vi "Drive Until Loss of Vision.vi"(11 "Distance Setpoint":dbl=56.0) -> (3 "ready to approach":bool=TRUE)   [LabVIEW 2016]
uses:
  Robot Values.vi
  Vision Global.vi
  <vilib>/addons/control/pid/pid.llb/PID (DBL).vi
  <vilib>/addons/control/pid/NI_PID_pid.lvlib
panel:
  in  "Baseline Power":dbl=0.5
  in  "Vision PID Gains":T1={"proportional gain (Kc)"=0.65, "integral time (Ti, min)"=0.0, "derivative time (Td, min)"=0.0} {"derivative time (Td, min)" format="%.3f"; "integral time (Ti, min)" format="%.3f"; "proportional gain (Kc)" format="%.3f"}
  in  "PID gains":T1={"proportional gain (Kc)"=1.0, "integral time (Ti, min)"=0.01, "derivative time (Td, min)"=0.0} {"derivative time (Td, min)" format="%.3f"; "integral time (Ti, min)" format="%.3f"; "proportional gain (Kc)" format="%.3f"}
  in  "Distance SP":dbl
  # "Disabled"
  # "Disabled"
  # "Enabled"
  # "original p 1 I .01"
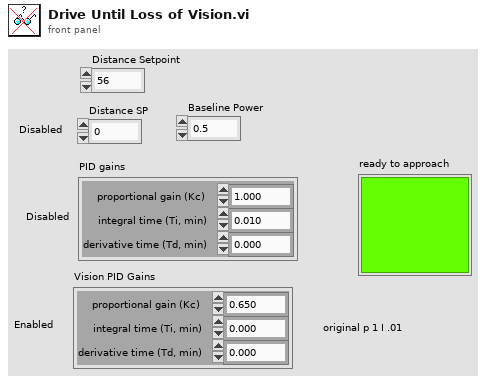
[diagram p1: front panel]
types:
  T1 = cluster{"proportional gain (Kc)":dbl, "integral time (Ti, min)":dbl, "derivative time (Td, min)":dbl}
  T2 = cluster{"Distance (ft)":dbl, "Score":dbl, "Normalized":cluster{"Center":cluster{dbl, dbl}, "Rectangle":cluster{"Numeric":dbl, "Numeric 2":dbl, "Numeric 3":dbl, "Numeric 5":dbl}}, "Pixels":cluster{"Center":cluster{dbl, dbl}, "Rectangle":cluster{"Numeric":dbl, "Numeric 2":dbl, "Numeric 3":dbl, "Numeric 5":dbl}}}
  T3 = typedef "Robot Values.ctl" = cluster{"Robot Drive":cluster{"Left Motor Power":dbl, "Right Motor Power":dbl, "Left Encoder Value":dbl, "Right Encoder Value":dbl, "High Gear?":bool, "PTO?":bool}, "Sensors":cluster{"Gyro Angle":u16, "Recalibrate Gyro":bool, "Reset Gyro":bool, "Ultrasonic":dbl}, "Shooter":cluster{"Prep Wheels":bool, "Shoot":bool, "Left Shooter Wheel Speed":dbl, "Wheels Moving":bool, "Shooter Prepped":bool, "Shooter RPS SP":dbl, "Shooting?":bool, "Left Shooter Wheel Power":dbl, "Right Shooter Wheel Power":dbl, "Acquisition Conveyor Power":dbl, "Hopper Beater Bar Power":dbl, "Filtered Left Shooter Speed":dbl, "Acquisition Motor Power":dbl, "Joystick Add":dbl}, "Robot States":cluster{"Drive mode":string, "Alliance":T4, "Position":T5}, "Gear":cluster{"Ejection Active":bool}}
  T4 = typedef "WPI_DriverStationAllianceInfo.ctl" = enum16{"Red", "Blue", "Invalid"}
  T5 = typedef "WPI_DriverStationPositionInfo.ctl" = enum16{"1", "2", "3"}
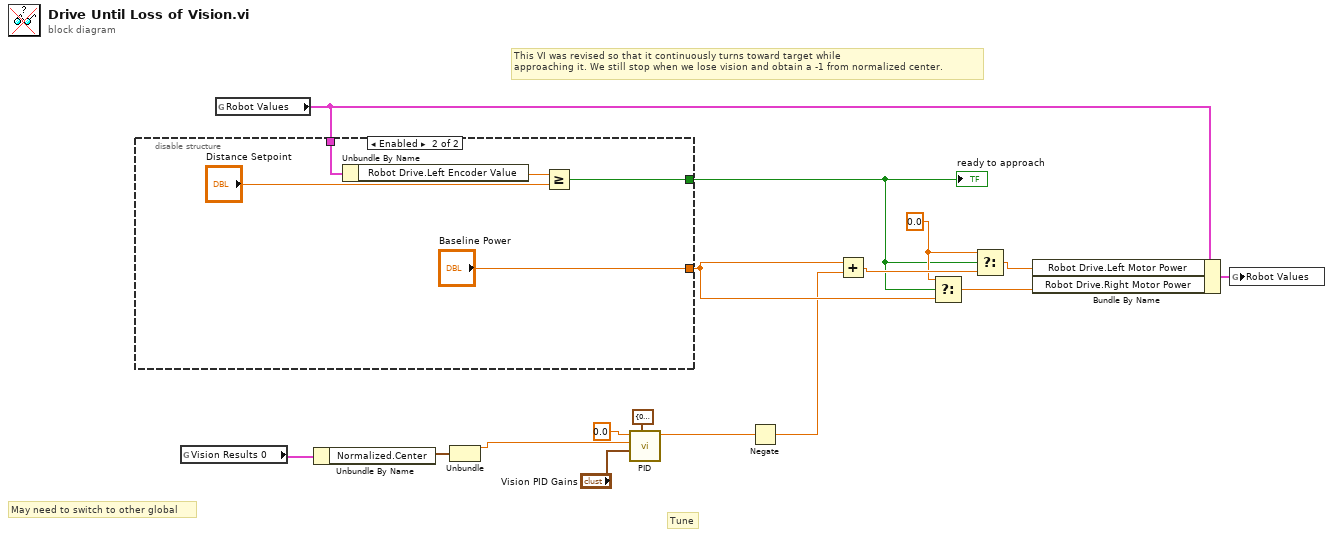
[diagram p0: block diagram]
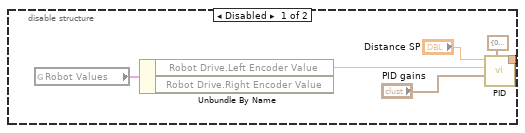
[diagram p2: hidden frame]
diagram:
  w7 = 0.0 ("t")
  # "This VI was revised so that it continuously turns toward target while \napproaching it. We still stop when we lose vision and obtain a -1 from normalized center."
  # "Tune"
  # "May need to switch to other global"
  n1 = global read "Vision Global.vi" "Vision Results 0"() -> (w15:T2)
  n2 = global read "Robot Values.vi" "Robot Values"() -> (w2:T3)
  n3 = disable-structure shown="Enabled" {
    disable-tunnel: [w18 "Baseline Power"] -> w10
    disable-tunnel: w2 -> [_ w26]
    disable-tunnel: [_ w23] -> w1
    frame Disabled {
      n4 = global read "Robot Values.vi" "Robot Values"() -> (w22:T3)
      n5 = Unbundle By Name(w22) -> ("Robot Drive.Left Encoder Value"=w19:dbl)  [unwired: 1 out]
      n6 = call-poly <vilib>:"PID.vi"("output range"=cluster{"output high":dbl, "output low":dbl} {"output high"=0.5, "output low"=-0.5}, "PID gains"="PID gains", "process variable"=w19, "setpoint"="Distance SP") -> ("output"=w18:dbl)  [unwired: 6 in, 1 out]
    }
    frame Enabled {
      n7 = Unbundle By Name(w26) -> ("Robot Drive.Left Encoder Value"=w25:dbl)
      n8 = Greater Or Equal?(x=w25, y="Distance Setpoint") -> (x >= y?=w23:bool)
    }
  }
  "ready to approach" <- w1
  n9 = Unbundle By Name(w15) -> ("Normalized.Center"=w14:cluster{dbl, dbl})
  n10 = Unbundle(w14) -> (w5:dbl)  [unwired: 1 out]
  n11 = call-poly <vilib>:"PID.vi"("output range"=cluster{"output high":dbl, "output low":dbl} {"output high"=0.2, "output low"=-0.2}, "PID gains"="Vision PID Gains", "process variable"=w5, "setpoint"=0.0) -> ("output"=w4:dbl)  [unwired: 6 in, 1 out]
  n12 = Negate(x=w4) -> (-x=w3:dbl)
  n13 = Add(x=w10, y=w3) -> (x+y=w9:dbl)
  n14 = Select(t=w7, s=w1, f=w10) -> (s? t:f=w6:dbl)
  n15 = Select(t=w7, s=w1, f=w9) -> (s? t:f=w8:dbl)
  n16 = Bundle By Name(cluster=w2, "Robot Drive.Left Motor Power"=w8, "Robot Drive.Right Motor Power"=w6) -> (w16:T3)
  n17 = global write "Robot Values.vi" "Robot Values"(w16) -> ()
